vi "inputoptical.vi"() -> ()   [LabVIEW 2009]
panel:
  in  "stop":bool
  out "Array":bool[](array[boolean])
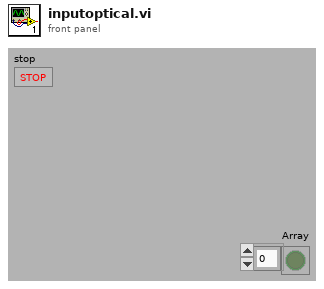
[diagram p1: front panel]
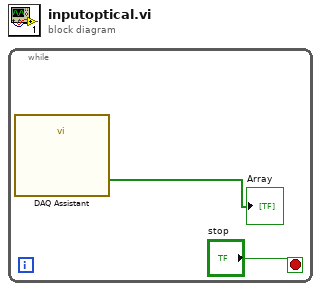
[diagram p0: block diagram]
diagram:
  n1 = while {
    stop <- "stop" stop-if-true
    n2 = call "DAQ Assistant"() -> ("data"=→"Array":bool[])  [unwired: 17 in, 2 out]
  }
